vi "ErrorProcessor_Template.vi"(8 "error in":errorcluster, 11 "error processor":refnum<class "ErrorProcessor.lvclass">) -> (0 "error out":errorcluster)   [LabVIEW 2013, in "CLM_ErrorHandler.lvlib"]
uses:
  CLM_ErrorHandler.lvlib
  ErrorProcessor/ErrorProcessor.lvclass
panel:
  in  "stop":bool
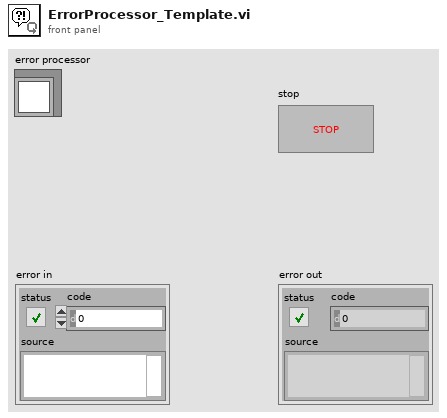
[diagram p1: front panel]
types:
  T1 = typedef "CLM_ErrorHandler.lvlib/ErrorMessage.ctl" = cluster{"error":errorcluster, "classification":string, "time reported":timestamp, "reporting process":string}
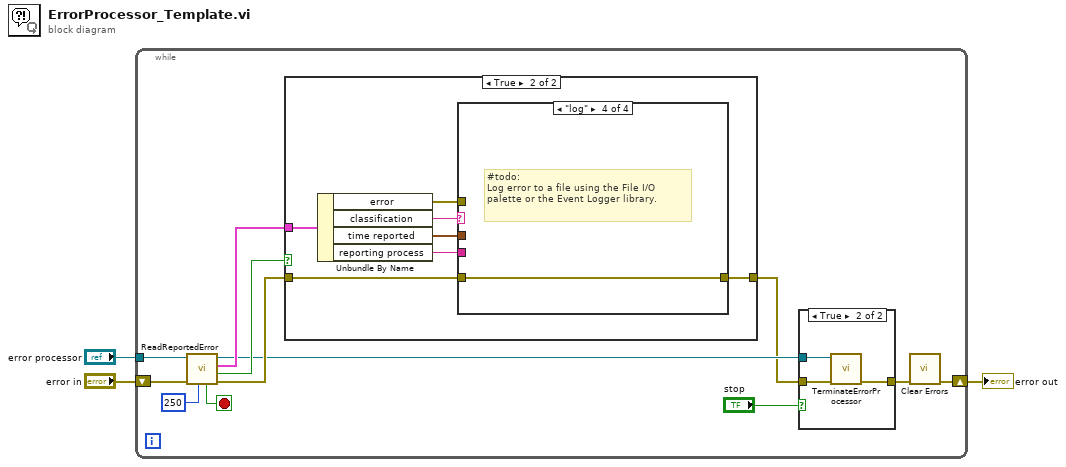
[diagram p0: block diagram]
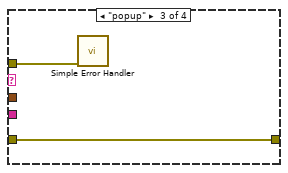
[diagram p6: hidden frame]
diagram:
  n1 = while {
    shift-right: [w5] -> w2
    shift-left: "error in" -> [w14]
    tunnel: "error processor" -> [w15]
    stop <- w12 stop-if-true
    n2 = call "ReadReportedError.vi"("timeout in ms (-1)"=250, "error in"=w14, "error processor in"=w15) -> ("error out"=w10:errorcluster, "error received?"=w11:bool, "error message"=w9:T1, "error processor out"=w8:refnum<class "ErrorProcessor.lvclass">, "terminate loop?"=w12:bool)  [unwired: 4 in]
    n3 = case shown="True" w11 {
      tunnel: w10 -> [w20 w25]
      tunnel: w9 -> [_ w27]
      tunnel: [w20 w21] -> w7
      frame False {
        # "No error received."
      }
      frame True {
        n4 = Unbundle By Name(w27) -> ("error"=w22:errorcluster, "classification"=w26:string, "time reported"=w23:timestamp, "reporting process"=w24:string)
        n5 = case shown="\"log\"" w26 {
          tunnel: w25 -> [w28 w29 w31 w32]
          tunnel: w24 -> [_ _ _ _]
          tunnel: w23 -> [_ _ _ _]
          tunnel: w22 -> [_ _ w30 _]
          tunnel: [w28 w29 w31 w32] -> w21
          frame Default {
          }
          frame "ignore" {
            # "Do nothing for errors classified as \"ignore\"."
          }
          frame "popup" {
            n6 = call <vilib>:"Simple Error Handler.vi"("error in (no error)"=w30) -> ()  [unwired: 4 in, 5 out]
          }
          frame "log" {
            # "#todo:\nLog error to a file using the File I/O palette or the Event Logger library."
          }
        }
      }
    }
    n7 = case shown="True" "stop" {
      tunnel: w8 -> [_ w19]
      tunnel: w7 -> [w16 w18]
      tunnel: [w16 w17] -> w4
      frame False {
      }
      frame True {
        n8 = call "TerminateErrorProcessor.vi"("error in"=w18, "error processor in"=w19) -> ("error out"=w17:errorcluster)  [unwired: 8 in, 1 out]
      }
    }
    n9 = call <vilib>:"Clear Errors.vi"("error in (no error)"=w4) -> ("error out"=w5:errorcluster)  [unwired: 6 in]
  }
  "error out" <- w2
